vi "SubVi.vi"() -> (2 "Mode":i32=1)   [LabVIEW 2020]
panel:
  in  "StableReadingIndic":u32 min=1 max=255 step=1
  in  "Accept":bool
  in  "Cancel":bool
  # "Введите пароль"
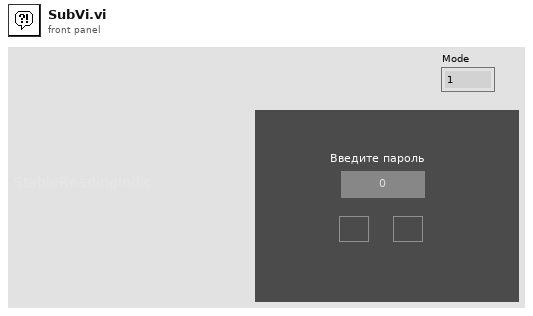
[diagram p1: front panel]
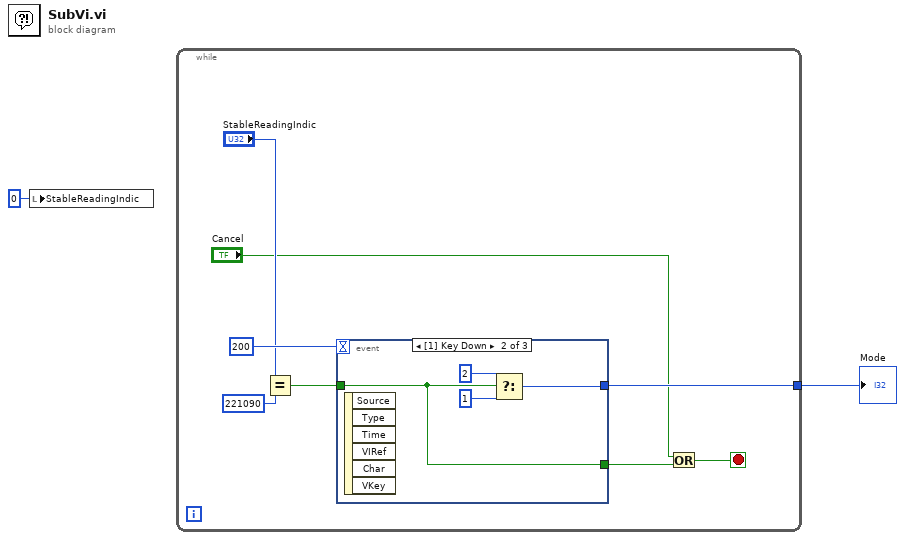
[diagram p0: block diagram]
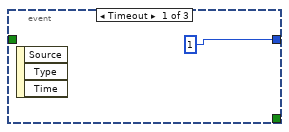
[diagram p2: hidden frame]
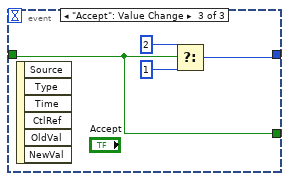
[diagram p3: hidden frame]
diagram:
  n1 = local write "StableReadingIndic"(u32 0 ("StableReadingIndic")) -> ()
  n2 = while {
    tunnel: [w6] -> w1
    stop <- w5 stop-if-true
    n3 = Equal?(x="StableReadingIndic", y=u32 221090) -> (x = y?=w7:bool)
    n4 = event shown="[1] Key Down" {
      selector: _ -> [_ _ _]
      dyn-events: _ -> [_ _ _]
      timeout: 200 -> [_ _ _]
      tunnel: w7 -> [_ w12 w16]
      tunnel: [1 w13 w17] -> w6
      tunnel: [_ w12 w16] -> w4
      event Timeout {
        n5 = event-data() -> ()  [unwired: 1 in, 3 out]
      }
      event Key Down {
        n6 = event-data() -> ()  [unwired: 1 in, 6 out]
        n7 = Select(t=2, s=w12, f=1) -> (s? t:f=w13:i32)
      }
      event "Accept": Value Change {
        n8 = event-data() -> ()  [unwired: 1 in, 6 out]
        n9 = Select(t=2, s=w16, f=1) -> (s? t:f=w17:i32)
      }
    }
    n10 = Or(x="Cancel", y=w4) -> (x .or. y?=w5:bool)
  }
  "Mode" <- w1
